vi "SetExtTrig.vi"   [LabVIEW 2014]
uses:
  ESLSCDLL.dll
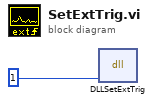
[diagram p0: block diagram]
diagram:
  n1 = dll-call lib="C:/Users/Gerhard/Documents/New64/lv/1cam/board.vis/ESLSCDLL.dll" fn="DLLSetExtTrig"("drv"=u32 1) -> ()  [unwired: 5 in, 2 out]
